vi "Read Results from processing.vi"(8 "error in":errorcluster, 11 "Temperature Controller Logic runtime in":refnum<class "Temperature Controller Logic runtime.lvclass">) -> (0 "error out":errorcluster, 2 "Results from processing":T1, 3 "Temperature Controller Logic runtime out":refnum<class "Temperature Controller Logic runtime.lvclass">)   [LabVIEW 2013, in "Temperature Controller Logic runtime.lvclass"]
uses:
  Temperature Controller Logic runtime.lvclass
  configuration/result data indices.ctl
  Temperature Controller Logic runtime.lvclass/Temperature Controller Logic runtime.ctl
  configuration/Temperature Controller Logic configuration.lvclass
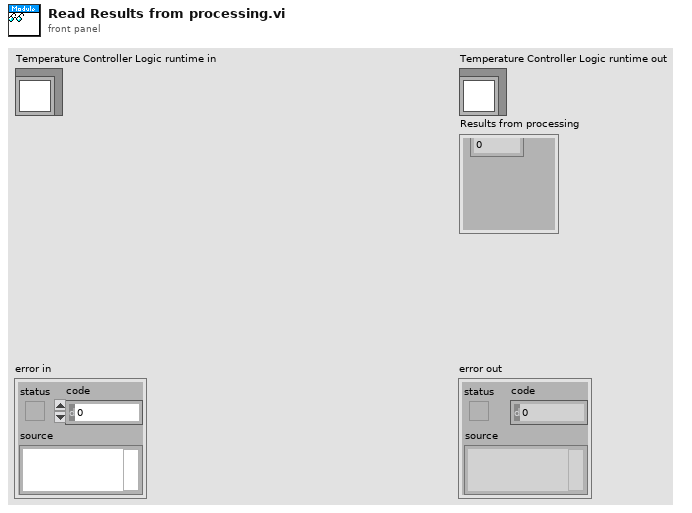
[diagram p1: front panel]
types:
  T1 = typedef "Temperature Controller Logic configuration.lvclass/result data indices.ctl" = cluster{"Double.fan":i32, "Double.lamp":i32, "U8.counter":i32}
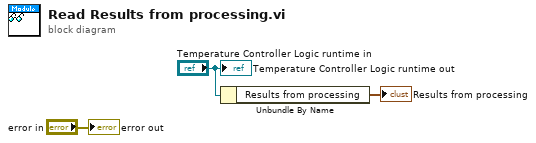
[diagram p0: block diagram]
diagram:
  n1 = Unbundle By Name("Temperature Controller Logic runtime in") -> ("Results from processing"=→"Results from processing":T1)
  "error out" <- "error in"
  "Temperature Controller Logic runtime out" <- "Temperature Controller Logic runtime in"
